vi "XY Plot.vi"(0 "X":dbl(slide) scale=-1.0..1.0, 1 "X array":dbl[](array[numeric]), 2 "Y array":dbl[](array[numeric]), 3 "Y":dbl(slide) scale=-1.0..1.0) -> (6 "XY Graph":cluster{"Y":dbl[], "Y":dbl[]}[](graph), 7 "X array":dbl[](array[numeric]), 8 "Y array":dbl[](array[numeric]), 9 "error out":errorcluster)   [LabVIEW 2014]
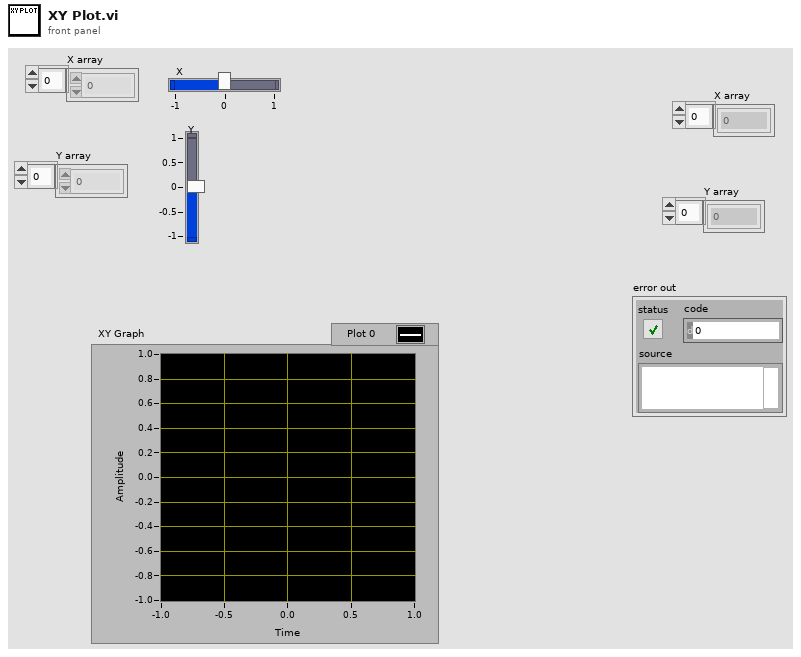
[diagram p1: front panel]
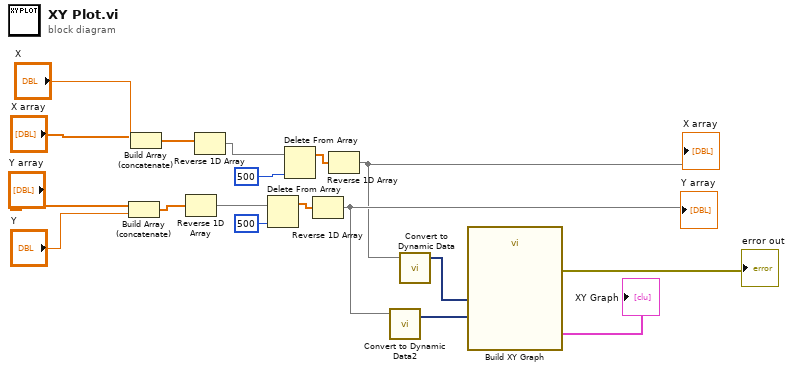
[diagram p0: block diagram]
diagram:
  n1 = Build Array (concatenate)("Y array", "Y") -> (w8:dbl[])
  n2 = Build Array (concatenate)("X array", "X") -> (w10:dbl[])
  n3 = Reverse 1D Array(array=w8) -> (reversed array=w7:dbl[])
  n4 = Reverse 1D Array(array=w10) -> (reversed array=w9:dbl[])
  n5 = Delete From Array(array=w7, index=500) -> (array with subset deleted=w6:dbl[])  [unwired: 1 in, 1 out]
  n6 = Delete From Array(array=w9, index=500) -> (array with subset deleted=w4:dbl[])  [unwired: 1 in, 1 out]
  n7 = Reverse 1D Array(array=w6) -> (reversed array=w5:dbl[])
  "Y array" <- w5
  n8 = Reverse 1D Array(array=w4) -> (reversed array=w3:dbl[])
  "X array" <- w3
  n9 = call "Convert to Dynamic Data2"("Array"=w5) -> ("Dynamic Data Type"=w13:dynamicdata)  [unwired: 3 in]
  n10 = call "Convert to Dynamic Data"("Array"=w3) -> ("Dynamic Data Type"=w12:dynamicdata)  [unwired: 3 in]
  n11 = call "Build XY Graph"("Y Input"=w13, "X Input"=w12) -> ("error out"=→"error out":errorcluster, "XY Graph"=→"XY Graph":cluster{"X":dbl[], "Y":dbl[]}[])  [unwired: 8 in]
